vi "Serial_Close.vi"(3 "error in (no error)":errorcluster) -> (0 "error out":errorcluster)   [LabVIEW 2009, in "Serial.lvlib"]
doc: "Closes the serial port VISA session and releases the semaphore reference. Should be called in the end of the program."
uses:
  Serial.lvlib
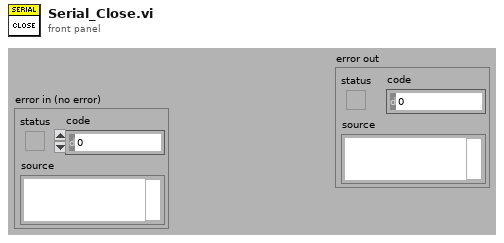
[diagram p1: front panel]
types:
  T1 = typedef "Semaphore RefNum" = refnum<k1>
  T2 = cluster{"VISA resource name":refnum<visa-resource-name>, "Semaphore":T1}
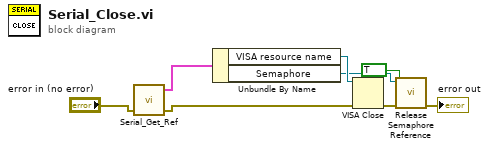
[diagram p0: block diagram]
diagram:
  n1 = call "Serial_Get_Ref.vi"("error in (no error)"="error in (no error)") -> ("error out"=w3:errorcluster, "Serial Ref"=w2:T2)  [unwired: 3 in]
  n2 = Unbundle By Name(w2) -> ("VISA resource name"=w8:refnum<visa-resource-name>, "Semaphore"=w7:T1)
  n3 = VISA Close(VISA resource name=w8, error in (no error)=w3) -> (error out=w6:errorcluster)
  n4 = call <vilib>:"Release Semaphore Reference.vi"("error in (no error)"=w6, "force destroy? (F)"=TRUE, "semaphore"=w7) -> ("error out"=→"error out":errorcluster)  [unwired: 7 in, 1 out]
